vi "GenerateVI_Icon.vi"(8 "error in (no error)":errorcluster, 11 "Text":T1) -> (0 "error out":errorcluster, 2 "Picture":picture, 3 "Icon.lvlclass out":refnum<class "Icon.lvclass">)   [LabVIEW 2017, in "MessageGen.lvlib"]
doc: "Basic example that shows how to set the Template Layer."
uses:
  <vilib>/addons/InsightCM/MessageBus/CodeGen/MessageGen.lvlib
  <vilib>/LabVIEW Icon API/lv_icon/Classes/Icon/Icon.lvclass
  <vilib>/LabVIEW Icon API/API_Text.ctl
  <vilib>/LabVIEW Icon API/LabVIEW Icon API.lvlib
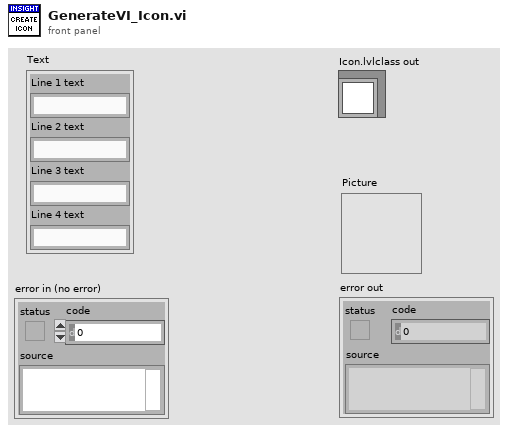
[diagram p1: front panel]
types:
  T1 = typedef "LabVIEW Icon API.lvlib/API_Text.ctl" = cluster{"Line 1 text":string, "Line 2 text":string, "Line 3 text":string, "Line 4 text":string}
  T2 = typedef "imagedata.ctl" = cluster{"image type":i32, "image depth":i32, "image":u8[], "mask":u8[], "colors":u32[], "Rectangle":cluster{"left":i16, "top":i16, "right":i16, "bottom":i16}}
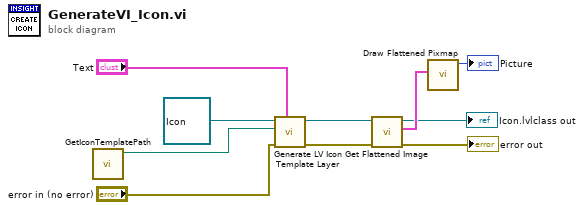
[diagram p0: block diagram]
diagram:
  n1 = call <vilib>:"GetIconTemplatePath.vi"() -> ("icon template"=w1:path)  [unwired: 11 in]
  n2 = call <vilib>:"Generate LV Icon Template Layer.vi"("Text"="Text", "error in (no error)"="error in (no error)", "Template path"=w1, "Icon.lvclass in"=refnum<class "Icon.lvclass"> refnum) -> ("error out"=w4:errorcluster, "Icon.lvclass out"=w3:refnum<class "Icon.lvclass">)  [unwired: 6 in]
  n3 = call <vilib>:"Get Flattened Image.vi"("error in (no error)"=w4, "lv_icon.lvlib:Icon.lvclass in"=w3) -> ("error out"=→"error out":errorcluster, "Color Image"=w8:T2, "lv_icon.lvlib:Icon.lvclass out"=→"Icon.lvlclass out":refnum<class "Icon.lvclass">)  [unwired: 6 in, 1 out]
  n4 = call <vilib>:"Draw Flattened Pixmap.vi"("image data"=w8) -> ("new picture"=→"Picture":picture)  [unwired: 8 in]
